vi "PlcDateTime.vi"() -> ()   [LabVIEW 2015]
uses:
  lib/Snap7.lvlib
panel:
  out "?":string
  in  "arbitrary":bool
  in  "sys":bool
  out "System Date/Time":timestamp
  in  "Arbitrary Date/Time":timestamp
  out "PLC Date/Time":timestamp
  in  "Error":i32
  in  "stop":bool
  out "Status":string
  in  "Slot":i32=2
  in  "Rack":i32
  in  "Address IP":string="192.168.1.12"
  # "Set System Date/Time"
  # "Set Arbitrary Date/Time"
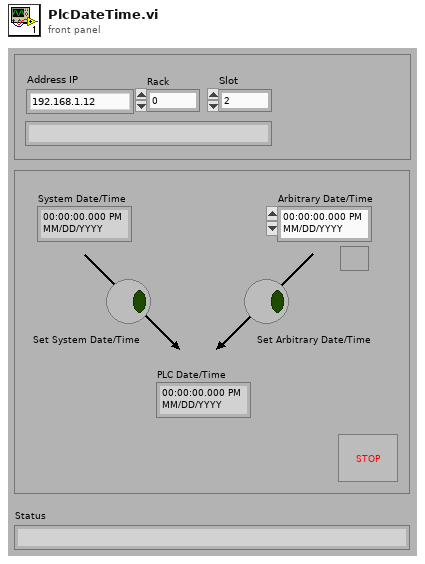
[diagram p1: front panel]
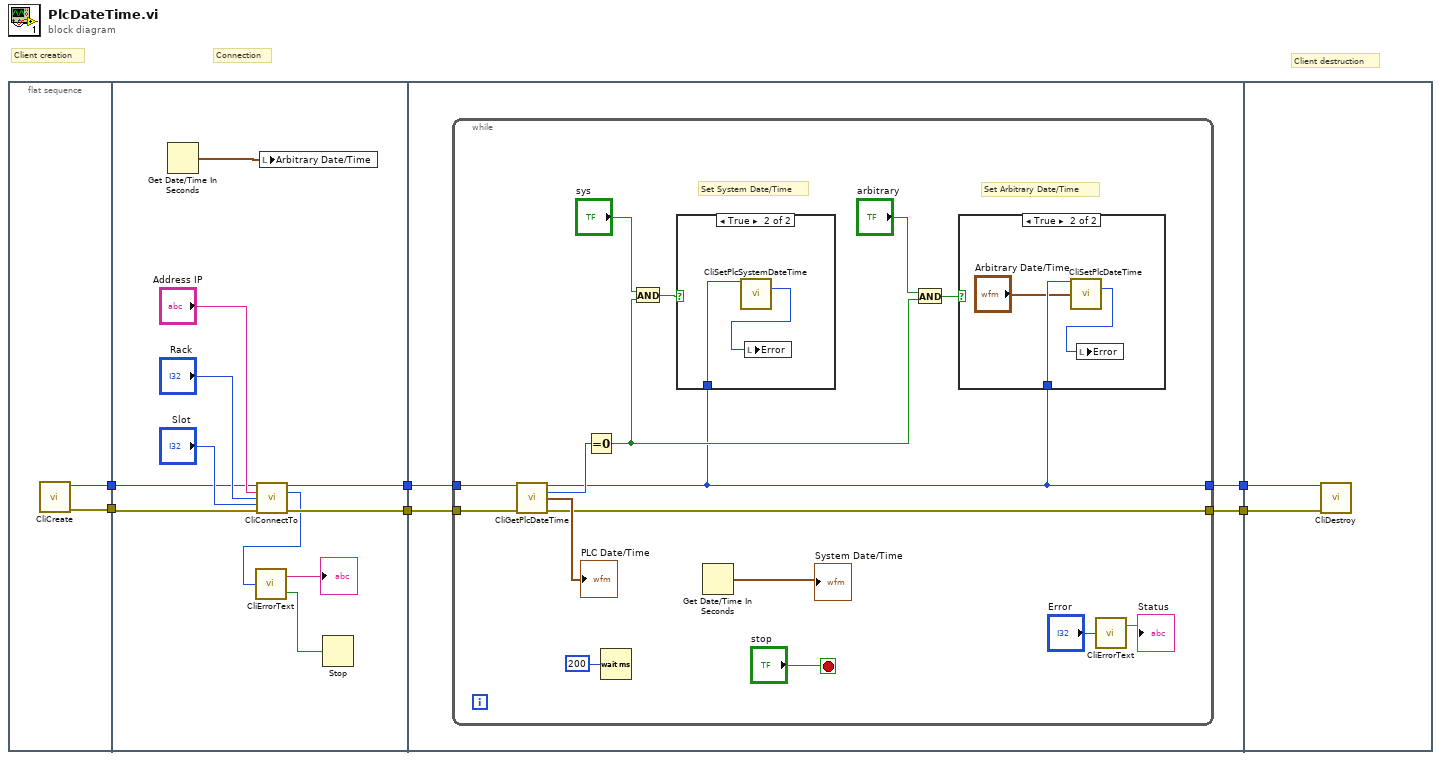
[diagram p0: block diagram]
diagram:
  # "Client destruction"
  # "Connection"
  # "Client creation"
  n1 = flat-sequence {
    tunnel: [w8] -> w4
    tunnel: [w7] -> w3
    tunnel: [w19] -> w6
    tunnel: [w13] -> w5
    tunnel: w4 -> [w15]
    tunnel: w3 -> [w14]
    tunnel: w5 -> [w23]
    tunnel: w6 -> [w22]
    tunnel: [w21] -> w2
    tunnel: [w20] -> w1
    tunnel: w2 -> [w46]
    tunnel: w1 -> [w45]
    frame #0 {
      n2 = call "CliCreate.vi"() -> ("ref out"=w8:u64, "error out"=w7:errorcluster)  [unwired: 14 in]
    }
    frame #1 {
      n3 = Get Date/Time In Seconds() -> (seconds since 1Jan1904=w12:timestamp)
      n4 = call "CliConnectTo.vi"("ref in"=w15, "Address"="Address IP", "Rack"="Rack", "Slot"="Slot", "error in (no error)"=w14) -> ("ref out"=w13:u64, "Result"=w9:i32, "error out"=w19:errorcluster)  [unwired: 8 in]
      n5 = call "CliErrorText.vi"("ErrNo"=w9) -> ("Error"=w10:bool, "ErrMessage"=→"?":string)
      n6 = local write "Arbitrary Date/Time"(w12) -> ()
      n7 = Stop(stop? (T)=w10) -> ()
    }
    frame #2 {
      n8 = while {
        tunnel: w23 -> [w38]
        tunnel: w22 -> [w37]
        tunnel: [w26] -> w21
        tunnel: [w35] -> w20
        stop <- "stop" stop-if-true
        # "Set Arbitrary Date/Time"
        # "Set System Date/Time"
        n9 = call "CliGetPlcDateTime.vi"("ref in"=w38, "error in (no error)"=w37) -> ("ref out"=w26:u64, "Result"=w32:i32, "DateTime"=→"PLC Date/Time":timestamp, "error out"=w35:errorcluster)  [unwired: 10 in]
        n10 = Equal To 0?(x=w32) -> (x = 0?=w30:bool)
        n11 = Wait (ms)(milliseconds to wait=u32 200 ("Loop Delay (ms)")) -> ()  [unwired: 1 out]
        n12 = And(x="sys", y=w30) -> (x .and. y?=w34:bool)
        n13 = case shown="True" w34 {
          tunnel: w26 -> [_ w44]
          frame False {
          }
          frame True {
            n14 = call "CliSetPlcSystemDateTime.vi"("ref in"=w44) -> ("Result"=w43:i32)  [unwired: 12 in, 2 out]
            n15 = local write "Error"(w43) -> ()
          }
        }
        n16 = Get Date/Time In Seconds() -> (seconds since 1Jan1904=→"System Date/Time":timestamp)
        n17 = And(x="arbitrary", y=w30) -> (x .and. y?=w29:bool)
        n18 = case shown="True" w29 {
          tunnel: w26 -> [_ w42]
          frame False {
          }
          frame True {
            n19 = call "CliSetPlcDateTime.vi"("ref in"=w42, "TimeStamp"="Arbitrary Date/Time") -> ("Result"=w40:i32)  [unwired: 11 in, 2 out]
            n20 = local write "Error"(w40) -> ()
          }
        }
        n21 = call "CliErrorText.vi"("ErrNo"="Error") -> ("ErrMessage"=→"Status":string)  [unwired: 1 out]
      }
    }
    frame #3 {
      n22 = call "CliDestroy.vi"("ref in"=w46, "error in (no error)"=w45) -> ()  [unwired: 13 in, 1 out]
    }
  }
